vi "Encoder Control Logic.vi"(8 "Prev Phase B (State Bit 1)":bool, 9 "Prev Phase A (State Bit 0)":bool, 10 "Phase B":bool, 11 "Phase A":bool) -> (1 "Count?":bool, 2 "Backward?":bool, 3 "Error Occurred?":bool)   [LabVIEW 2017]
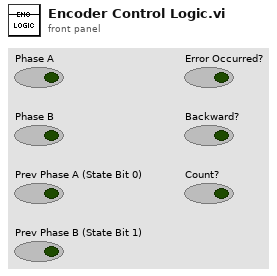
[diagram p1: front panel]
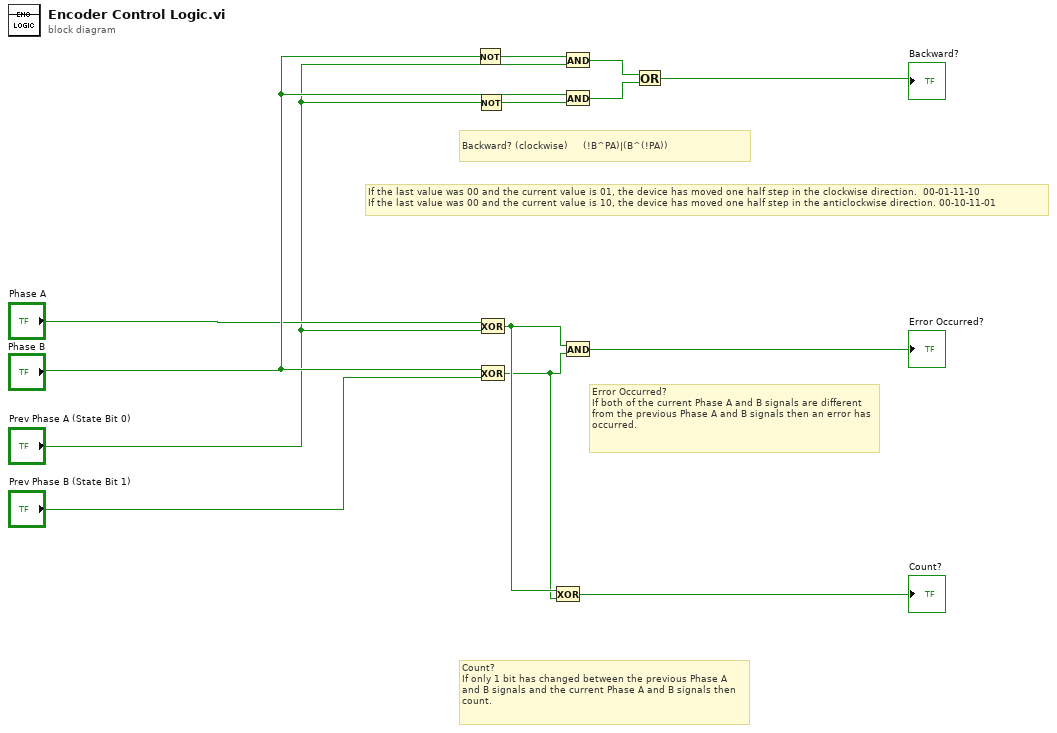
[diagram p0: block diagram]
diagram:
  # "If the last value was 00 and the current value is 01, the device has moved one half step in the clockwise direction.  00-01-11-10 \nIf the last value was 00 and the current value is 10, the device has moved one half step in the anticlockwise direction. 00-10-11-01"
  # "Backward? (clockwise)     (!B^PA)|(B^(!PA))"
  # "Count? \nIf only 1 bit has changed between the previous Phase A and B signals and the current Phase A and B signals then count."
  # "Error Occurred?\nIf both of the current Phase A and B signals are different from the previous Phase A and B signals then an error has occurred."
  n1 = Not(x="Phase B") -> (.not. x?=w12:bool)
  n2 = Not(x="Prev Phase A (State Bit 0)") -> (.not. x?=w11:bool)
  n3 = Exclusive Or(1:"Prev Phase A (State Bit 0)", 2:"Phase A") -> (0:w2:bool)
  n4 = Exclusive Or(1:"Prev Phase B (State Bit 1)", 2:"Phase B") -> (0:w1:bool)
  n5 = Exclusive Or(1:w1, 2:w2) -> (0:→"Count?":bool)
  n6 = And(x=w12, y="Prev Phase A (State Bit 0)") -> (x .and. y?=w9:bool)
  n7 = And(x="Phase B", y=w11) -> (x .and. y?=w10:bool)
  n8 = And(x=w2, y=w1) -> (x .and. y?=→"Error Occurred?":bool)
  n9 = Or(x=w9, y=w10) -> (x .or. y?=→"Backward?":bool)
